vi "Time to subscribe.vi"(8 "error in (no error)":errorcluster, 11 "Measure Object in":refnum<class "Measure Object.lvclass">) -> (0 "error out":errorcluster, 3 "Measure Object out":refnum<class "Measure Object.lvclass">)   [LabVIEW 2015, in "Measure Object.lvclass"]
uses:
  Measure Object.lvclass
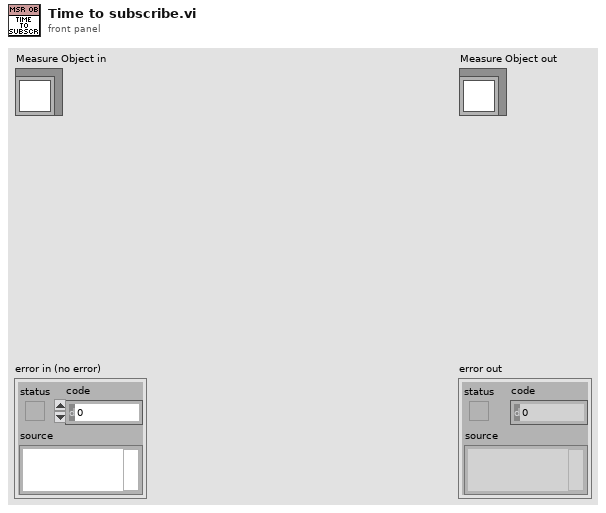
[diagram p1: front panel]
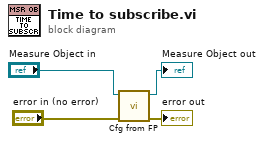
[diagram p0: block diagram]
diagram:
  n1 = call-dynamic "Cfg from FP.vi"("error in (no error)"="error in (no error)", "Measure Object in"="Measure Object in") -> ("error out"=→"error out":errorcluster, "Measure Object out"=→"Measure Object out":refnum<class "Measure Object.lvclass">)  [unwired: 8 in]
